vi "加标回收启动 (子VI).vi"(11 "启动参数":T1(ring)=enum."CODCr") -> (0 "error out":T2={"status"=FALSE, "代码"=4, "source"=""} caption="错误输出" {"代码" items=["执行成功"=1, "执行失败，但不知道原因"=2, "命令请求条件错误"=3, "通讯超时"=4, "系统繁忙不能执行"=5, "系统故障"=6, "没有数据"=100]})   [LabVIEW 2016, in "MB SLAVE.lvlib"]
uses:
  MB SLAVE.lvlib
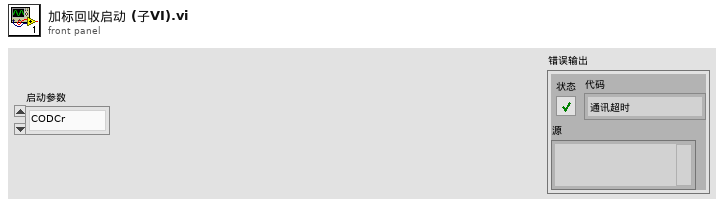
[diagram p1: front panel]
types:
  T1 = enum16{"未选择", "CODMn", "氨氮", "总磷", "总氮", "CODCr"}
  T2 = cluster{"status":bool, "代码":u16, "source":string}
  T3 = typedef "测试子流程.ctl" = enum16{"加标回收（启动采配水）", "加标回收（不启动采配水）", "水样测试（启动采配水）", "水样测试（不启动采配水）", "平行样测试（启动采配水）", "平行样测试（不启动采配水）", "集成干预测试"}
  T4 = typedef "质控slave id.ctl" = enum16{"null", "氨氮", "总磷", "总氮", "CODMn", "CODCr", "氟化物"}
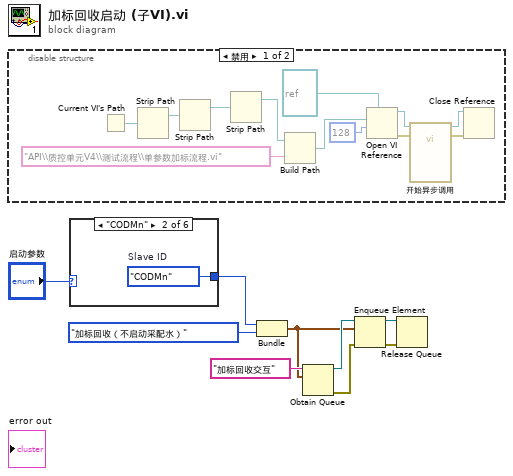
[diagram p0: block diagram]
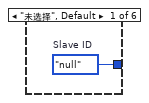
[diagram p3: hidden frame]
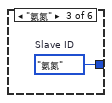
[diagram p4: hidden frame]
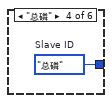
[diagram p5: hidden frame]
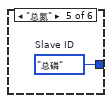
[diagram p6: hidden frame]
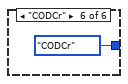
[diagram p7: hidden frame]
diagram:
  n1 = disable-structure shown="禁用" {
    frame Disabled {
      n2 = Current VI's Path() -> (path=w21:path)
      n3 = Strip Path(path=w21) -> (stripped path=w12:path)  [unwired: 1 out]
      n4 = Strip Path(path=w12) -> (stripped path=w11:path)  [unwired: 1 out]
      n5 = Strip Path(path=w11) -> (stripped path=w19:path)  [unwired: 1 out]
      n6 = Build Path(base path=w19, name or relative path="API\\质控单元V4\\测试流程\\单参数加标流程.vi" ("名称或相对路径")) -> (appended path=w13:path)
      n7 = Open VI Reference(type specifier VI Refnum (for type only)=refnum<vi> refnum, vi path=w13, options=128 ("选项")) -> (vi reference=w15:refnum<vi>, error out=w16:errorcluster)  [unwired: 3 in]
      n8 = call-by-ref "开始异步调用"(reference=w15, error in=w16) -> (reference out=w17:refnum<vi>, error out=w18:errorcluster)  [unwired: 12 in]
      n9 = Close Reference(reference=w17, error in (no error)=w18) -> ()  [unwired: 1 out]
    }
    frame Enabled {
    }
  }
  n10 = case shown="\"CODMn\"" "启动参数" {
    tunnel: [w22 w23 w24 w25 w26 质控slave_id."CODCr" ("Slave ID")] -> w3
    frame "未选择", Default {
      w22 = 质控slave_id."null"  # Slave ID
    }
    frame "CODMn" {
      w23 = 质控slave_id."CODMn"  # Slave ID
    }
    frame "氨氮" {
      w24 = 质控slave_id."氨氮"  # Slave ID
    }
    frame "总磷" {
      w25 = 质控slave_id."总磷"  # Slave ID
    }
    frame "总氮" {
      w26 = 质控slave_id."总磷"  # Slave ID
    }
    frame "CODCr" {
    }
  }
  n11 = Bundle("Slave ID"=w3, "流程参数"=测试子流程."加标回收（不启动采配水）") -> (w2:cluster{"Slave ID":T4, "流程参数":T3})  [unwired: 1 in]
  n12 = Obtain Queue(name (unnamed)="加标回收交互" ("名称（未命名）"), element data type=w2) -> (queue out=w7:refnum<queue>, error out=w6:errorcluster)  [unwired: 3 in, 1 out]
  n13 = Enqueue Element(queue=w7, element=w2, error in (no error)=w6) -> (queue out=w5:refnum<queue>, error out=w4:errorcluster)  [unwired: 1 in, 1 out]
  n14 = Release Queue(queue=w5, error in (no error)=w4) -> ()  [unwired: 1 in, 3 out]
